vi "Init.vi"(8 "error in (no error)":errorcluster, 10 "Instrument String":variant, 11 "NI Thermo in":refnum<class "NI Thermo.lvclass">) -> (0 "error out":errorcluster, 2 "Found?":bool=TRUE, 3 "NI Thermo out":refnum<class "NI Thermo.lvclass">)   [LabVIEW 2025, in "Thermo.lvlib" / "NI Thermo.lvclass"]
uses:
  NI Thermo.lvclass
  C:/Users/Public/Documents/Sandia National Labs/TSS Plugin/CEF.lvlibp/Node/CEF_Node.lvclass
  Thermo Channel/Thermo Channel.lvclass
  Thermo Channel configuration/Thermo Channel configuration.lvclass
  C:/Users/Public/Documents/Sandia National Labs/TSS Plugin/Abstract Engine.lvlibp/Plugin/Abstract/Channel configuration/Channel configuration.lvclass
  NI Thermo.lvclass/NI Thermo.ctl
  Thermo Channel configuration/Read Thermo Channel.vi
  Users/Public/Documents/Sandia National Labs/TSS Plugin/CEF.lvlibp/Node/ReadChildren.vi
  Users/Public/Documents/Sandia National Labs/TSS Plugin/Abstract Engine.lvlibp/Plugin/Abstract/Channel configuration/Read Channel Setting.vi
  Users/Public/Documents/Sandia National Labs/TSS Plugin/CEF.lvlibp/Node/CEF_Node.lvclass
  Users/Public/Documents/Sandia National Labs/TSS Plugin/CEF.lvlibp/serializable configuration/CEF_serializable configuration.lvclass
  <vilib>/DAQmx/create/channels.llb/DAQmx Create Channel (AI-Temperature-Thermocouple).vi
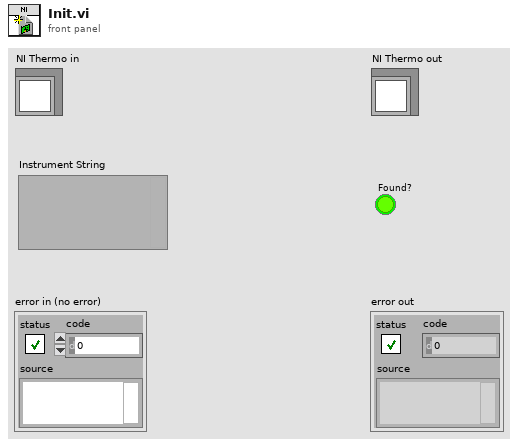
[diagram p1: front panel]
types:
  T1 = typedef "Abstract Engine.lvlibp/Channel configuration.lvclass/Default Channel.ctl" = cluster{"Address":string, "SW Alias":string, "Enabled":bool, "Type":string, "Description":string}
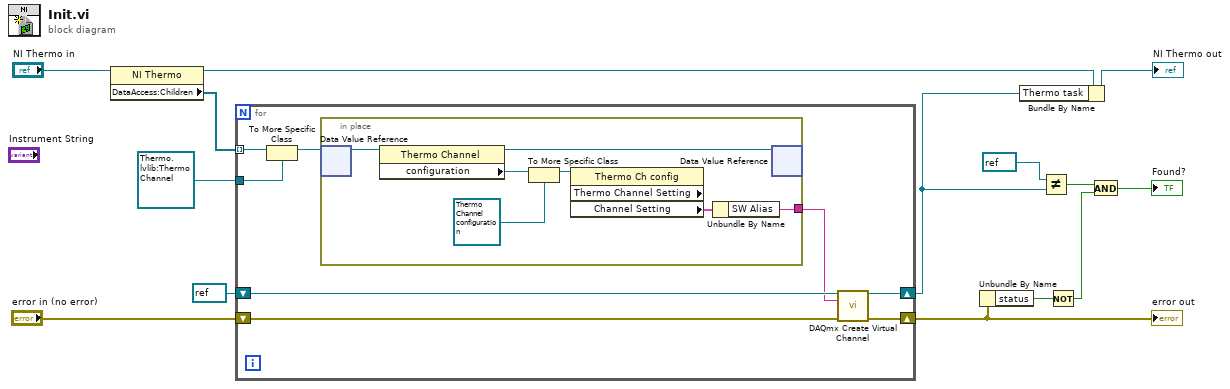
[diagram p0: block diagram]
diagram:
  n1 = property class="NI Thermo"(reference="NI Thermo in") -> (reference out=w12:refnum<class "NI Thermo.lvclass">, "DataAccess:Children"=w11:refnum<data-value>[])  [unwired: 1 in, 1 out]
  n2 = for {
    shift-right: [w22] -> w4
    shift-left: "error in (no error)" -> [w20]
    shift-right: [w21] -> w3
    shift-left: refnum<k21> refnum ("task out") -> [w19]
    tunnel: w11 -> [w18] mode=indexing
    tunnel: refnum<data-value> refnum ("data value reference") -> [w16]
    n3 = To More Specific Class(target class=w16, reference=w18) -> (specific class reference=w17:refnum<data-value>)  [unwired: 1 in, 1 out]
    n4 = in-place {
      in-place-border: [w27] -> w15
      # "Initialize the front panel controls when loaded"
      n5 = in-place-dvr #1(w17) -> (w28:refnum<class "Thermo Channel.lvclass">)  [unwired: 1 out]
      n6 = property class="Thermo Channel"(reference=w28) -> (reference out=w29:refnum<class "Thermo Channel.lvclass">, "configuration"=w26:refnum<class "CEF_serializable configuration.lvclass">)  [unwired: 1 in, 1 out]
      n7 = To More Specific Class(target class=refnum<class "Thermo Channel configuration.lvclass"> refnum ("Thermo.lvlib:Thermo Ch config"), reference=w26) -> (specific class reference=w25:refnum<class "Thermo Channel configuration.lvclass">)  [unwired: 1 in, 1 out]
      n8 = property class="Thermo Ch config" props=["Thermo Channel Setting", "Channel Setting"](reference=w25) -> ("Channel Setting"=w24:T1)  [unwired: 1 in, 3 out]
      n9 = Unbundle By Name(w24) -> ("SW Alias"=w27:string)
      n10 = in-place-dvr #1(w29) -> ()  [unwired: 2 out]
    }
    n11 = call-poly <vilib>:"DAQmx Create Virtual Channel.vi"("task in"=w19, "physical channels"=w15, "error in"=w20) -> ("task out"=w21:refnum<k21>, "error out"=w22:errorcluster)  [unwired: 11 in]
  }
  "error out" <- w4
  n12 = Unbundle By Name(w4) -> ("status"=w5:bool)
  n13 = Bundle By Name(cluster=w12, "Thermo task"=w3) -> (→"NI Thermo out":refnum<class "NI Thermo.lvclass">)
  n14 = Not Equal?(x=refnum<k21> refnum, y=w3) -> (x != y?=w7:bool)
  n15 = Not(x=w5) -> (.not. x?=w6:bool)
  n16 = And(x=w7, y=w6) -> (x .and. y?=→"Found?":bool)
